vi "username and password.vi"() -> ()   [LabVIEW 2020]
uses:
  2a1c4dbf-cb47-40d8-9944-75d56e6dffa3.vi
  e3e54044-086a-4766-8ea5-0eb672b2c677.vi
  <vilib>/Utility/file.llb/Read Delimited Spreadsheet (string).vi
  <vilib>/Comparison/Equal/Equal Functor/Equal Functor.lvclass
panel:
  out "s? t:f 2":string
  in  "String 2":string
  in  "String":string
  out "s? t:f":string
  in  "false":string
  in  "true":string
  in  "password":string
  in  "username":string
  in  "file path (dialog if empty)":path
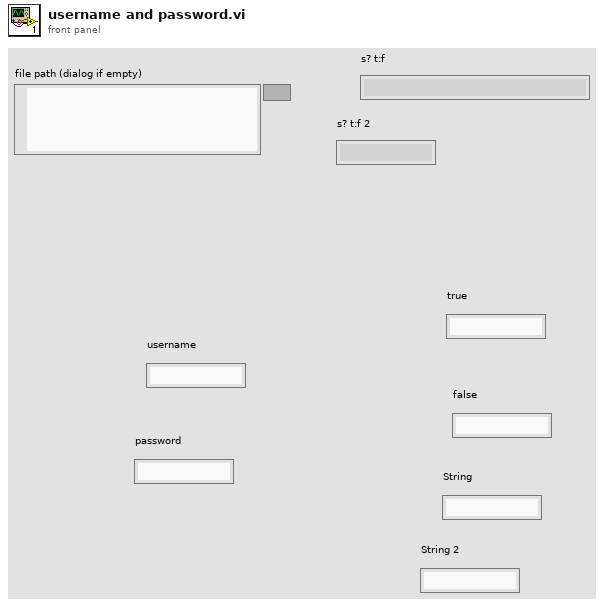
[diagram p1: front panel]
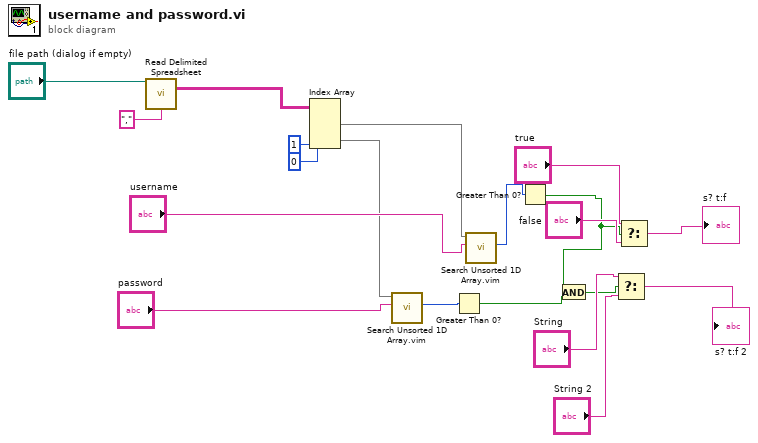
[diagram p0: block diagram]
diagram:
  n1 = call-poly <vilib>:"Read Delimited Spreadsheet.vi"("file path (dialog if empty)"="file path (dialog if empty)", "delimiter (\\t)"="," ("delimiter (\\t)")) -> ("all rows"=w19:string[][])  [unwired: 8 in, 5 out]
  n2 = Index Array(array=w19, index (col) #1=0 ("disabled index (col)"), index (col) #2=1 ("index (col)")) -> (element #1=w6:string[], element #2=w8:string[])  [unwired: 2 in]
  n3 = call "Search Unsorted 1D Array.vim"("element"="password", "unsorted 1D array"=w8) -> ("index of element"=w3:i32)  [unwired: 9 in]
  n4 = Greater Than 0?(x=w3) -> (x > 0?=w2:bool)
  n5 = call "Search Unsorted 1D Array.vim"("element"="username", "unsorted 1D array"=w6) -> ("index of element"=w5:i32)  [unwired: 9 in]
  n6 = Greater Than 0?(x=w5) -> (x > 0?=w4:bool)
  n7 = And(x=w4, y=w2) -> (x .and. y?=w1:bool)
  n8 = Select(t="String", s=w1, f="String 2") -> (s? t:f=→"s? t:f 2":string)
  n9 = Select(t="true", s=w4, f="false") -> (s? t:f=→"s? t:f":string)
